vi "arrange waveforms.vi"(1 "data":waveform(dbl)[](array[waveform])) -> (0 "Waveforms":T1)   [LabVIEW 2013]
uses:
  Controls/arranged waveforms.ctl
  Controls/waveform display.ctl
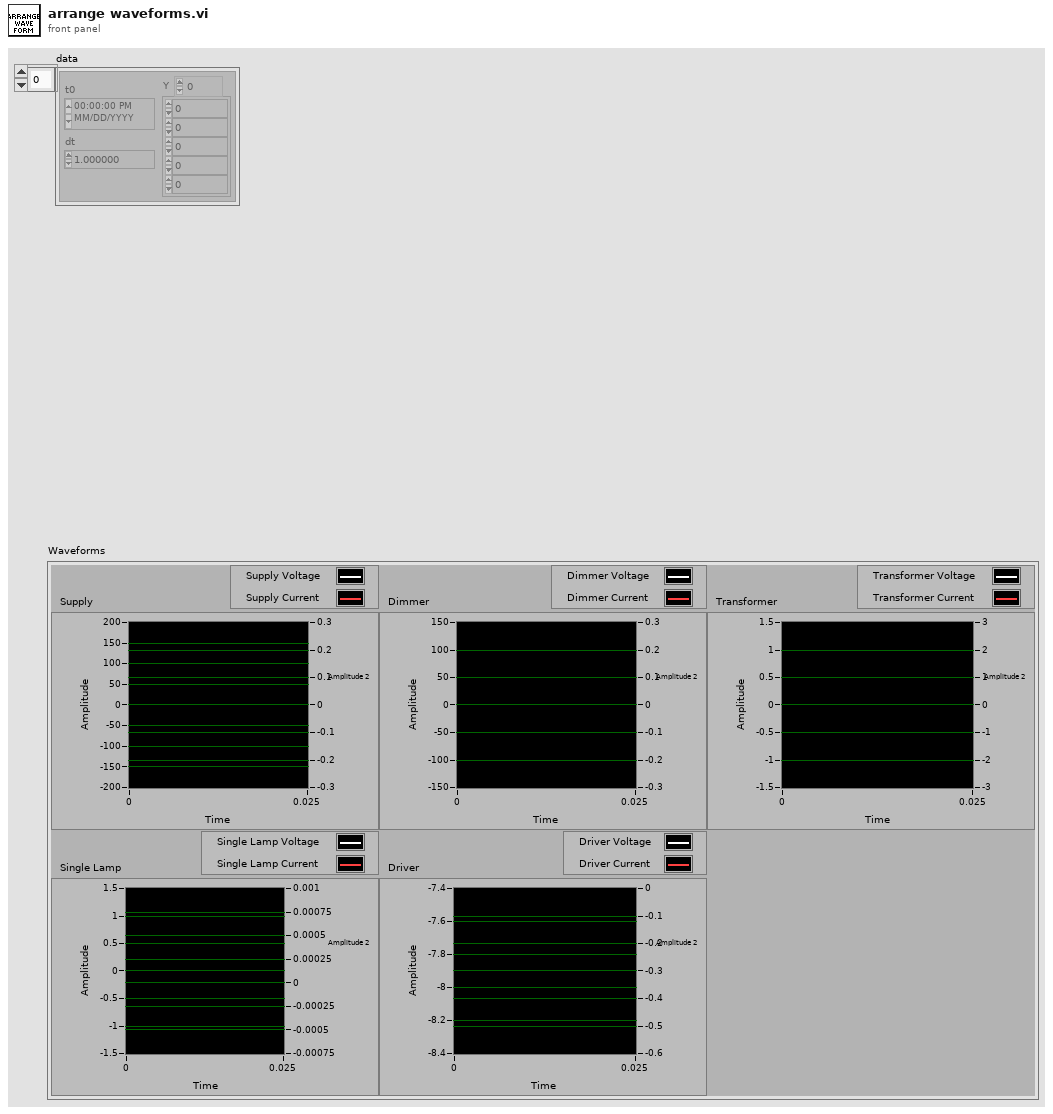
[diagram p1: front panel]
types:
  T1 = typedef "arranged waveforms.ctl" = cluster{"Supply":T2, "Dimmer":T2, "Transformer":T2, "Single Lamp":T2, "Driver":T2}
  T2 = typedef "waveform display.ctl" = waveform(dbl)[]
  T3 = cluster{waveform(dbl)[], waveform(dbl)[], waveform(dbl)[], waveform(dbl)[], waveform(dbl)[]}
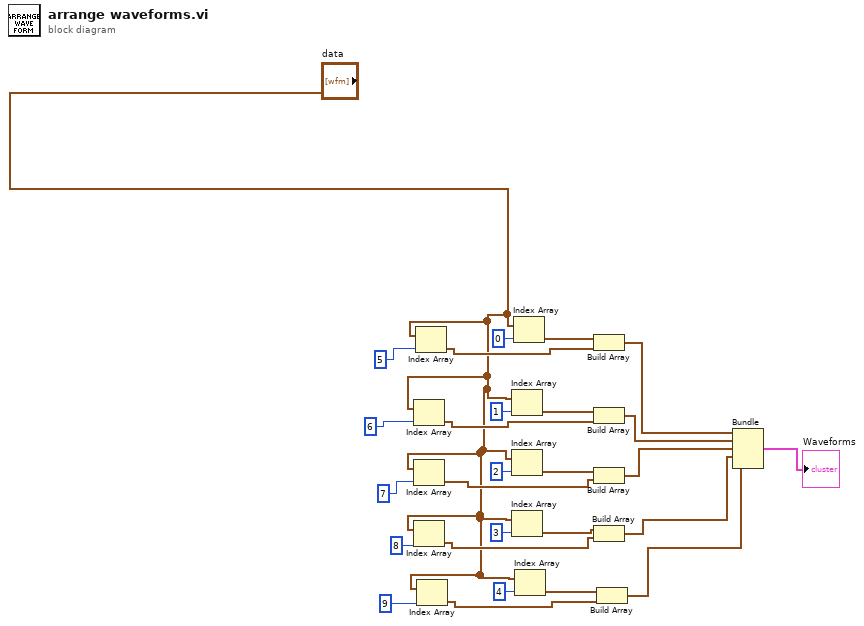
[diagram p0: block diagram]
diagram:
  n1 = Index Array(array="data", index=6) -> (element=w26:waveform(dbl))
  n2 = Index Array(array="data", index=7) -> (element=w25:waveform(dbl))
  n3 = Index Array(array="data", index=8) -> (element=w24:waveform(dbl))
  n4 = Index Array(array="data", index=5) -> (element=w27:waveform(dbl))
  n5 = Index Array(array="data", index=9) -> (element=w23:waveform(dbl))
  n6 = Index Array(array="data", index=1) -> (element=w15:waveform(dbl))
  n7 = Index Array(array="data", index=2) -> (element=w14:waveform(dbl))
  n8 = Index Array(array="data", index=3) -> (element=w13:waveform(dbl))
  n9 = Index Array(array="data", index=0) -> (element=w16:waveform(dbl))
  n10 = Index Array(array="data", index=4) -> (element=w12:waveform(dbl))
  n11 = Build Array(w16, w27) -> (w6:waveform(dbl)[])
  n12 = Build Array(w15, w26) -> (w5:waveform(dbl)[])
  n13 = Build Array(w14, w25) -> (w4:waveform(dbl)[])
  n14 = Build Array(w13, w24) -> (w3:waveform(dbl)[])
  n15 = Build Array(w12, w23) -> (w2:waveform(dbl)[])
  n16 = Bundle(w6, w5, w4, w3, w2) -> (→"Waveforms":T3)  [unwired: 1 in]
